vi "Interface Write.vi"(8 "error in":errorcluster, 9 "timeout":i32=10000, 10 "data":u8[](array[numeric]), 11 "TCP interface in":refnum<class "TCP Interface.lvclass">) -> (0 "error out":errorcluster, 1 "timed out?":bool, 3 "TCP interface out":refnum<class "TCP Interface.lvclass">)   [LabVIEW 2021, in "TCP Interface.lvclass"]
doc: "Writes to the established TCP connection stored in the class."
uses:
  TCP Interface.lvclass
  TCP Interface.lvclass/TCP Interface.ctl
  <vilib>/Utility/error.llb/Clear Errors.vi
  TCP Shared Components/TCP Shared Components.lvlib
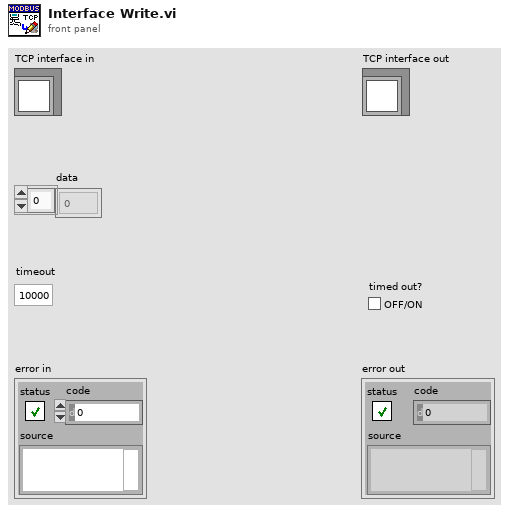
[diagram p1: front panel]
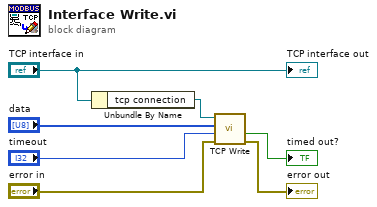
[diagram p0: block diagram]
diagram:
  n1 = Unbundle By Name("TCP interface in") -> ("tcp connection"=w1:refnum<k5>)
  n2 = call "TCP Write.vi"("error in"="error in", "timeout"="timeout", "data"="data", "connection ID"=w1) -> ("error out"=→"error out":errorcluster, "timed out?"=→"timed out?":bool)  [unwired: 6 in]
  "TCP interface out" <- "TCP interface in"
